vi "exercise1.vi"() -> ()   [LabVIEW 2021]
panel:
  in  "stop":bool
  in  "Keep Previous Locations":bool
  out "2D Picture":picture
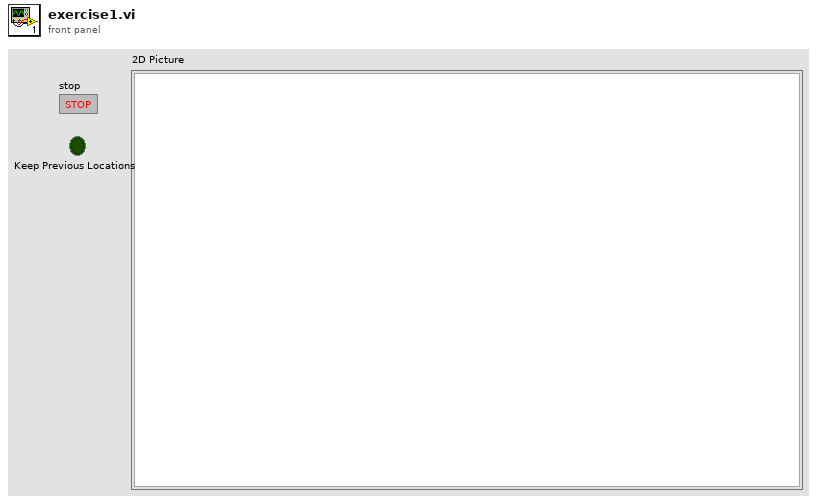
[diagram p1: front panel]
types:
  T1 = cluster{"Width":u16, "Style":enum32{"Solid", "Dash", "Dot", "DashDot", "DashDotDot"}}
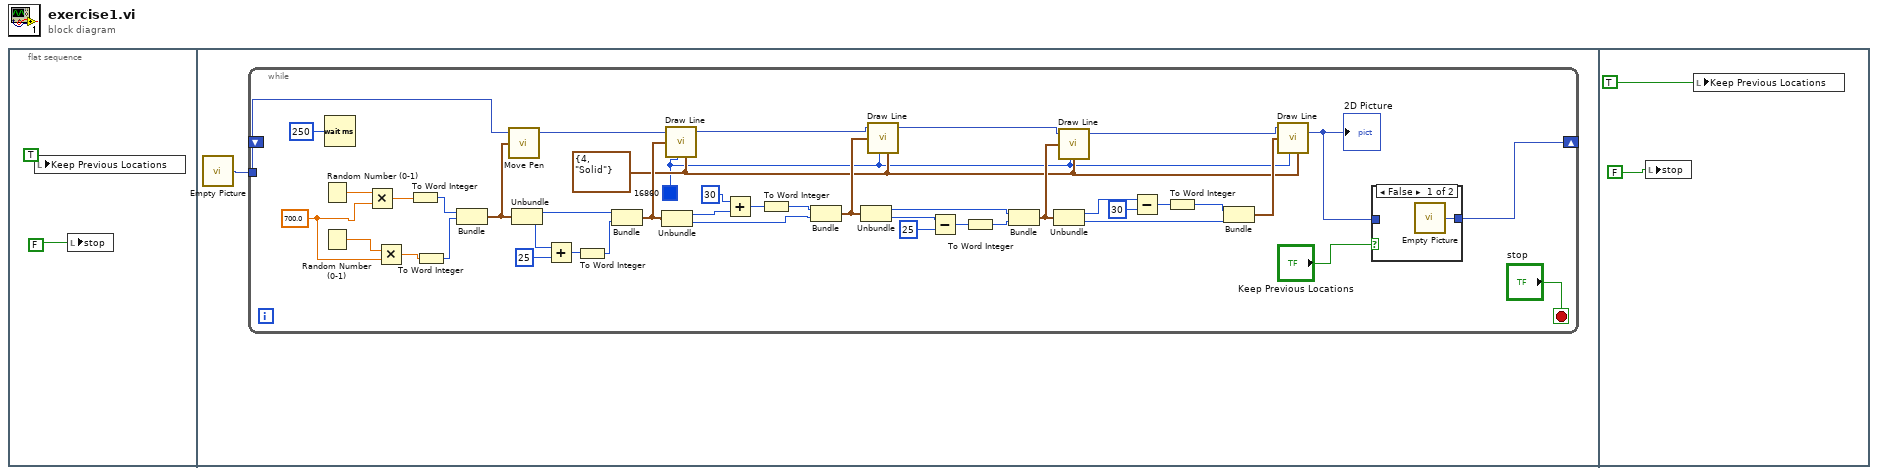
[diagram p0: block diagram]
diagram:
  n1 = flat-sequence {
    frame #0 {
      n2 = local write "Keep Previous Locations"(TRUE) -> ()
      n3 = local write "stop"(FALSE) -> ()
    }
    frame #1 {
      n4 = call "Empty Picture"() -> ("empty picture"=w3:picture)
      n5 = while {
        tunnel: w3 -> [w34]
        shift-right: [w6] -> _
        shift-left: _ -> [_]
        stop <- "stop" stop-if-true
        w7 = u32 16860 ("color(black)")
        w8 = T1 {"Width"=4, "Style"=enum."Solid"} ("pen")
        w42 = 700.0 ("y")
        n6 = Random Number (0-1)() -> (number: 0 to 1=w46:dbl)
        n7 = Random Number (0-1)() -> (number: 0 to 1=w45:dbl)
        n8 = Wait (ms)(milliseconds to wait=u32 250) -> ()  [unwired: 1 out]
        n9 = Multiply(x=w46, y=w42) -> (x*y=w43:dbl)
        n10 = Multiply(x=w45, y=w42) -> (x*y=w44:dbl)
        n11 = To Word Integer(number=w43) -> (16bit integer=w41:i16)
        n12 = To Word Integer(number=w44) -> (16bit integer=w40:i16)
        n13 = Bundle(w41, w40) -> (w35:cluster{i16, i16})  [unwired: 1 in]
        n14 = call <vilib>:"Move Pen.vi"("new position"=w35, "picture"=w34) -> ("new picture"=w13:picture)  [unwired: 3 in]
        n15 = Unbundle(w35) -> (w33:i16, w37:i16)
        n16 = Add(x=w37, y=i16 25) -> (x+y=w39:i16)
        n17 = To Word Integer(number=w39) -> (16bit integer=w38:i16)
        n18 = Bundle(w33, w38) -> (w32:cluster{i16, i16})  [unwired: 1 in]
        n19 = Unbundle(w32) -> (w31:i16, w27:i16)
        n20 = call <vilib>:"Draw Line.vi"("picture"=w13, "end point"=w32, "color(black)"=w7, "pen"=w8) -> ("new picture"=w12:picture)  [unwired: 5 in]
        n21 = Add(x=i16 30, y=w31) -> (x+y=w29:i16)
        n22 = To Word Integer(number=w29) -> (16bit integer=w28:i16)
        n23 = Bundle(w28, w27) -> (w26:cluster{i16, i16})  [unwired: 1 in]
        n24 = Unbundle(w26) -> (w21:i16, w25:i16)
        n25 = call <vilib>:"Draw Line.vi"("picture"=w12, "end point"=w26, "color(black)"=w7, "pen"=w8) -> ("new picture"=w11:picture)  [unwired: 5 in]
        n26 = Subtract(x=w25, y=i16 25) -> (x-y=w23:i16)
        n27 = To Word Integer(number=w23) -> (16bit integer=w22:i16)
        n28 = Bundle(w21, w22) -> (w20:cluster{i16, i16})  [unwired: 1 in]
        n29 = Unbundle(w20) -> (w19:i16, w15:i16)
        n30 = call <vilib>:"Draw Line.vi"("picture"=w11, "end point"=w20, "color(black)"=w7, "pen"=w8) -> ("new picture"=w10:picture)  [unwired: 5 in]
        n31 = Subtract(x=w19, y=i16 30) -> (x-y=w17:i16)
        n32 = To Word Integer(number=w17) -> (16bit integer=w16:i16)
        n33 = Bundle(w16, w15) -> (w14:cluster{i16, i16})  [unwired: 1 in]
        n34 = call <vilib>:"Draw Line.vi"("picture"=w10, "end point"=w14, "color(black)"=w7, "pen"=w8) -> ("new picture"=w5:picture)  [unwired: 5 in]
        "2D Picture" <- w5
        n35 = case shown="False" "Keep Previous Locations" {
          tunnel: [w48 w49] -> w6
          tunnel: w5 -> [_ w49]
          frame False {
            n36 = call "Empty Picture"() -> ("empty picture"=w48:picture)
          }
          frame True {
          }
        }
      }
    }
    frame #2 {
      n37 = local write "stop"(FALSE) -> ()
      n38 = local write "Keep Previous Locations"(TRUE) -> ()
    }
  }
